vi "motor run execution.vi"(8 "error in":errorcluster, 10 "data":T3, 11 "Refnum Cluster Motor":T1) -> (0 "error out":errorcluster, 2 "Motor TextLog":string, 3 "Motor Log":string[][](array[string]))   [LabVIEW 2022 SP3]
uses:
  7f3f7f10-a4f1-45dc-94b5-7ca3060defcc.vi
  3e648d45-6e5c-4607-959b-4bd81591d8b7.vi
  3b4dbe33-a398-4ae1-98f2-0f6a12eff476.vi
  f93c375e-c4a4-4129-880d-4f6f32d70360.vi
  42315686-0e40-4c30-95d1-eb6a4dfe8554.vi
  62005152-647d-4142-ac27-8e0444444e4d.vi
  720007ab-8e7a-4def-9525-68d42a256be9.vi
  5550de12-40e6-485b-bfc0-db9a801049c2.vi
  3894978a-308b-403e-95e7-56de26c9271f.vi
  71392560-3ac6-4d43-9930-287395f3e7a2.vi
  pectus/control/Param Epics Cluster.ctl
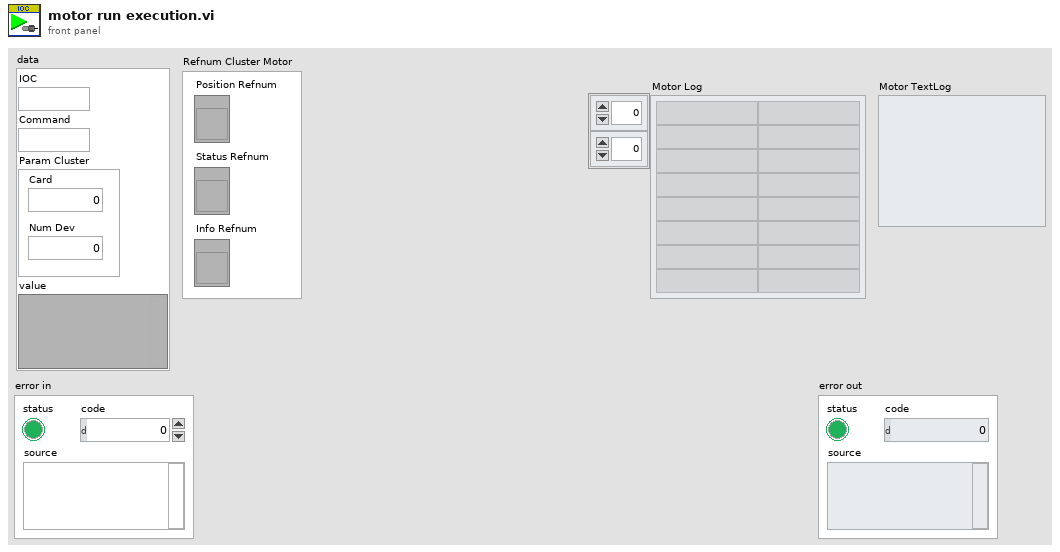
[diagram p1: front panel]
types:
  T1 = cluster{"Position Refnum":refnum<vi>, "Status Refnum":refnum<vi>, "Info Refnum":refnum<vi>}
  T2 = typedef "Param Epics Cluster.ctl" = cluster{"Card":u16, "Num Dev":u16}
  T3 = cluster{"IOC":string, "Command":string, "Param Cluster":T2, "value":variant}
  T4 = typedef "epics value.ctl" = cluster{"Record":string, "Value Out":variant}
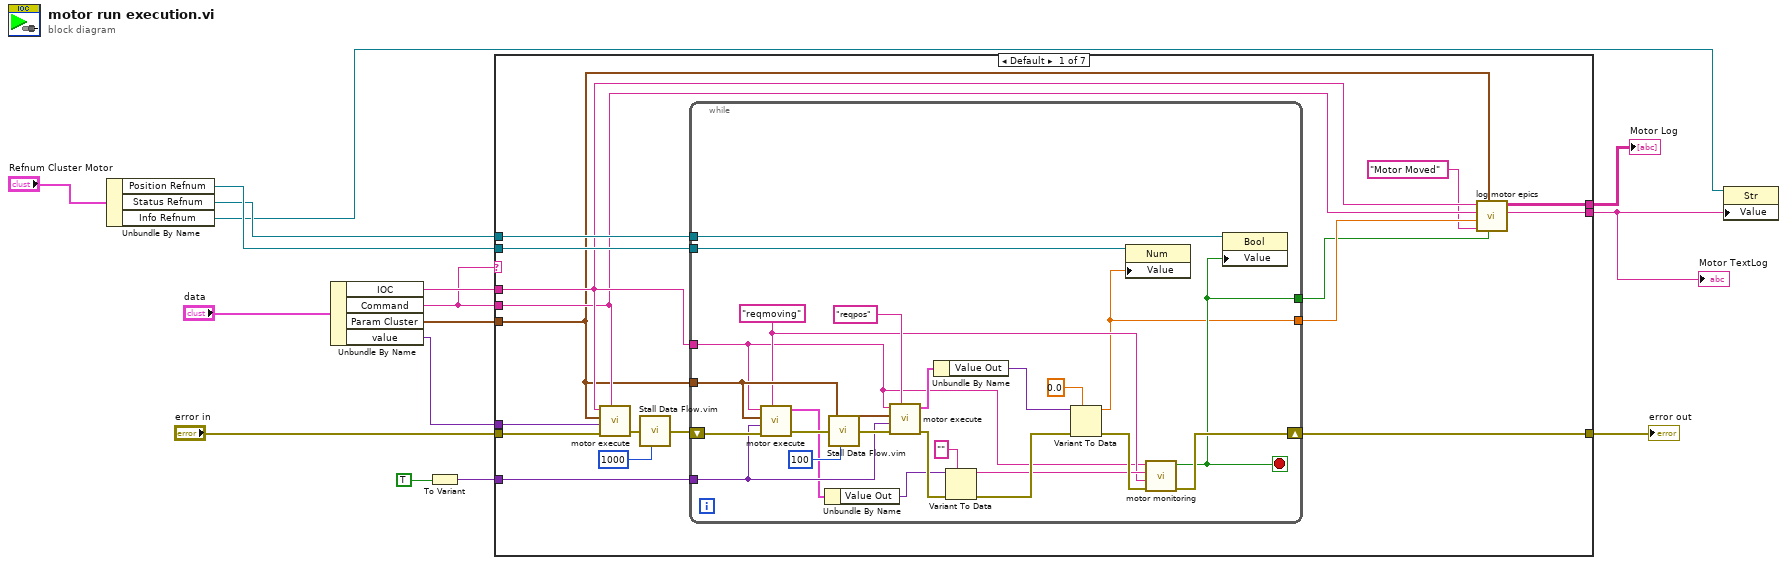
[diagram p0: block diagram]
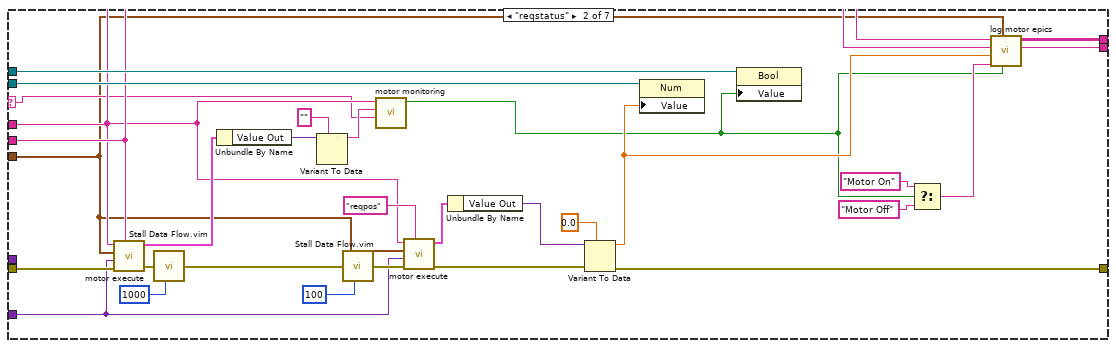
[diagram p2: hidden frame]
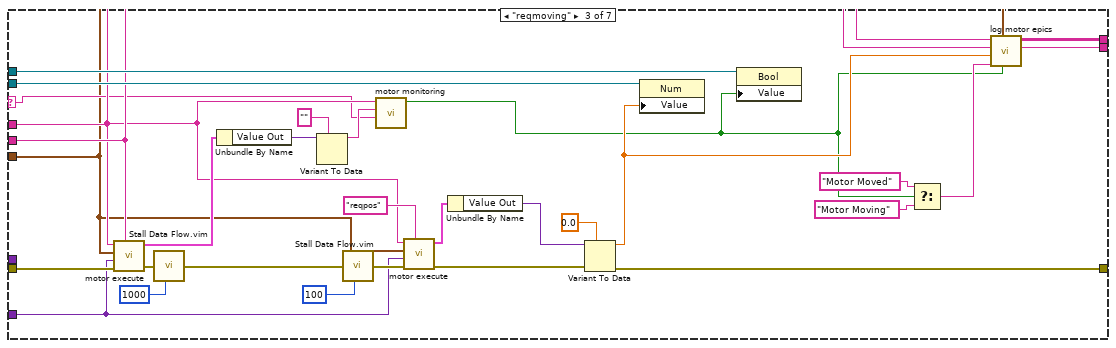
[diagram p3: hidden frame]
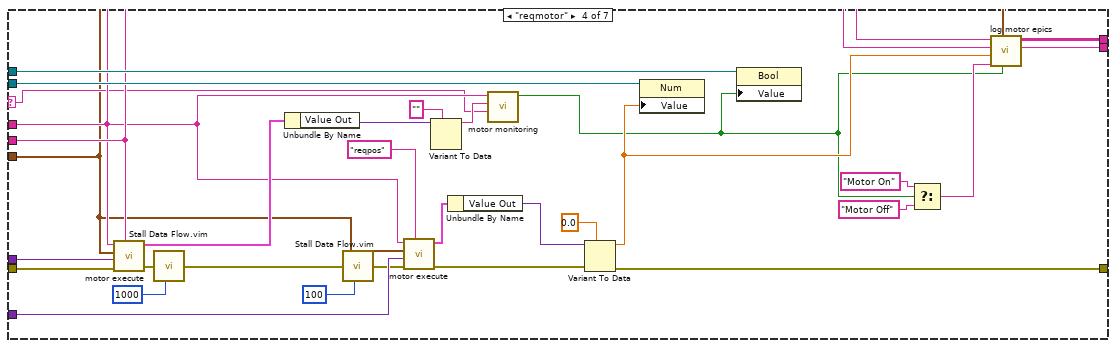
[diagram p4: hidden frame]
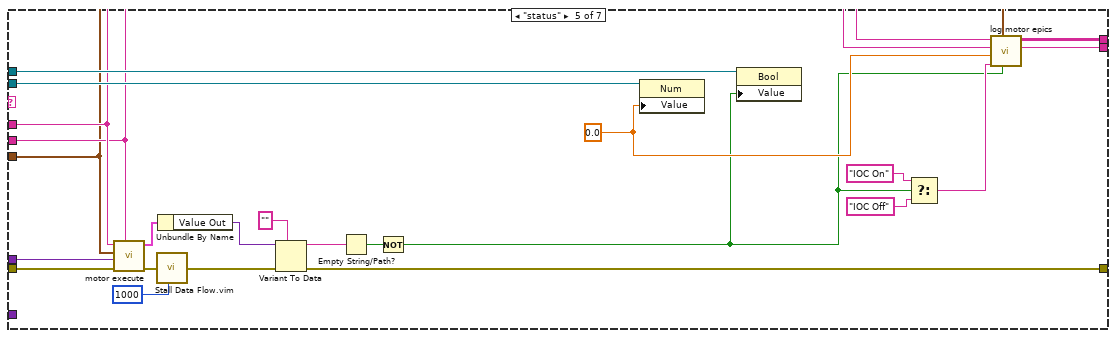
[diagram p5: hidden frame]
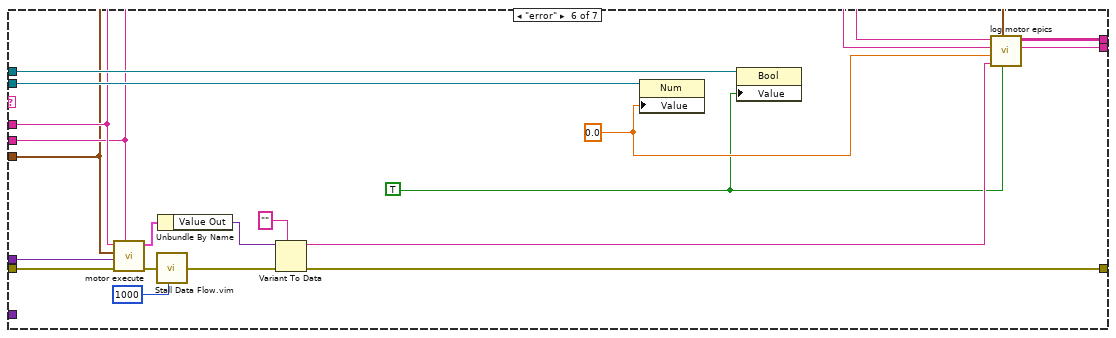
[diagram p6: hidden frame]
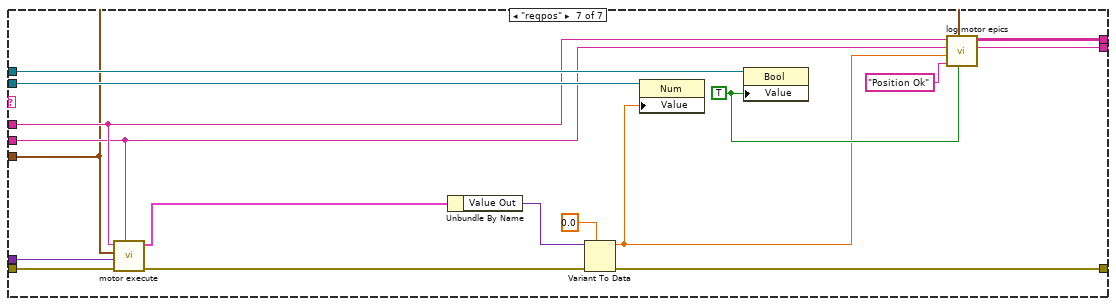
[diagram p7: hidden frame]
diagram:
  n1 = Unbundle By Name("Refnum Cluster Motor") -> ("Position Refnum"=w5:refnum<vi>, "Status Refnum"=w4:refnum<vi>, "Info Refnum"=w1:refnum<vi>)
  n2 = Unbundle By Name("data") -> ("IOC"=w13:string, "Command"=w7:string, "Param Cluster"=w14:T2, "value"=w11:variant)
  n3 = To Variant(anything=TRUE) -> (Variant=w15:variant)
  n4 = case shown="Default" w7 {
    selector: w7 -> [_ w59 w89 w118 _ _ _]
    tunnel: w15 -> [w29 w63 w93 w144 _ _ _]
    tunnel: w14 -> [w16 w57 w87 w117 w148 w171 w190]
    tunnel: w13 -> [w23 w62 w92 w120 w163 w182 w194]
    tunnel: w11 -> [w28 _ _ w143 w167 w186 w205]
    tunnel: w7 -> [w20 w78 w108 w137 w161 w180 w193]
    tunnel: "error in" -> [w27 w83 w113 w142 w166 w185 w204]
    tunnel: [w26 w82 w112 w141 w158 w177 w203] -> w8
    tunnel: w5 -> [w25 w81 w111 w140 w165 w184 w202]
    tunnel: w4 -> [w24 w80 w110 w139 w164 w183 w201]
    tunnel: [w19 w77 w107 w136 w160 w179 w197] -> w3
    tunnel: [w18 w76 w106 w135 w159 w178 w196] -> w2
    frame Default {
      n5 = call "motor execute.vi"("Command Motor"=w20, "error in"=w27, "Value"=w28, "Param Cluster"=w16, "IOC"=w23) -> ("error out"=w30:errorcluster)  [unwired: 3 in, 3 out]
      n6 = call "Stall Data Flow.vim"("value in"=w30, "milliseconds to wait"=u32 1000) -> ("value out"=w31:errorcluster)  [unwired: 1 out]
      n7 = while {
        shift-right: [w39] -> w26
        shift-left: w31 -> [w56]
        tunnel: w23 -> [w35]
        tunnel: w16 -> [w50]
        tunnel: w29 -> [w52]
        tunnel: w25 -> [w41]
        tunnel: w24 -> [w36]
        tunnel: [w34] -> w21
        tunnel: [w33] -> w22
        stop <- w34 stop-if-true
        w37 = "reqmoving"
        n8 = call "motor execute.vi"("Command Motor"=w37, "error in"=w56, "Value"=w52, "Param Cluster"=w50, "IOC"=w35) -> ("error out"=w55:errorcluster, "Data Value Out"=w43:T4)  [unwired: 3 in, 2 out]
        n9 = Unbundle By Name(w43) -> ("Value Out"=w42:variant)
        n10 = call "Stall Data Flow.vim"("value in"=w55, "milliseconds to wait"=u32 100) -> ("value out"=w53:errorcluster)  [unwired: 1 out]
        n11 = call "motor execute.vi"("Command Motor"="reqpos", "error in"=w53, "Value"=w52, "Param Cluster"=w50, "IOC"=w35) -> ("error out"=w46:errorcluster, "Data Value Out"=w47:T4)  [unwired: 3 in, 2 out]
        n12 = Unbundle By Name(w47) -> ("Value Out"=w49:variant)
        n13 = Variant To Data(error in=w46, type="", Variant=w42) -> (data=w38:string, error out=w45:errorcluster)
        n14 = Variant To Data(error in=w45, type=0.0, Variant=w49) -> (data=w33:dbl, error out=w40:errorcluster)
        n15 = property on="Property Node" class="Num"(reference=w41, "Value"=w33) -> ()  [unwired: 1 in, 2 out]
        n16 = call "motor monitoring.vi"("error in"=w40, "record"=w37, "Value"=w38, "IOC"=w35) -> ("error out"=w39:errorcluster, "Moved"=w34:bool)  [unwired: 6 in]
        n17 = property on="Property Node" class="Bool"(reference=w36, "Value"=w34) -> ()  [unwired: 1 in, 2 out]
      }
      n18 = call "log motor epics.vi"("status"=w21, "Param Cluster"=w16, "Info"="Motor Moved", "Position"=w22, "Command"=w20, "IOC"=w23) -> ("Motor TextLog"=w18:string, "Motor Log"=w19:string[][])  [unwired: 4 in]
    }
    frame "reqstatus" {
      n19 = call "motor execute.vi"("Command Motor"=w78, "error in"=w83, "Value"=w63, "Param Cluster"=w57, "IOC"=w62) -> ("error out"=w84:errorcluster, "Data Value Out"=w64:T4)  [unwired: 3 in, 2 out]
      n20 = call "Stall Data Flow.vim"("value in"=w84, "milliseconds to wait"=u32 1000) -> ("value out"=w85:errorcluster)  [unwired: 1 out]
      n21 = Unbundle By Name(w64) -> ("Value Out"=w65:variant)
      n22 = Variant To Data(type="", Variant=w65) -> (data=w60:string)  [unwired: 1 in, 1 out]
      n23 = call "Stall Data Flow.vim"("value in"=w85, "milliseconds to wait"=u32 100) -> ("value out"=w71:errorcluster)  [unwired: 1 out]
      n24 = call "motor monitoring.vi"("record"=w59, "Value"=w60, "IOC"=w62) -> ("Moved"=w58:bool)  [unwired: 7 in, 1 out]
      n25 = call "motor execute.vi"("Command Motor"="reqpos", "error in"=w71, "Value"=w63, "Param Cluster"=w57, "IOC"=w62) -> ("error out"=w66:errorcluster, "Data Value Out"=w67:T4)  [unwired: 3 in, 2 out]
      n26 = Unbundle By Name(w67) -> ("Value Out"=w69:variant)
      n27 = Variant To Data(error in=w66, type=0.0, Variant=w69) -> (data=w79:dbl, error out=w82:errorcluster)
      n28 = property on="Property Node" class="Num"(reference=w81, "Value"=w79) -> ()  [unwired: 1 in, 2 out]
      n29 = property on="Property Node" class="Bool"(reference=w80, "Value"=w58) -> ()  [unwired: 1 in, 2 out]
      n30 = Select(t="Motor On" ("Info"), s=w58, f="Motor Off" ("Info")) -> (s? t:f=w73:string)
      n31 = call "log motor epics.vi"("status"=w58, "Param Cluster"=w57, "Info"=w73, "Position"=w79, "Command"=w78, "IOC"=w62) -> ("Motor TextLog"=w76:string, "Motor Log"=w77:string[][])  [unwired: 4 in]
    }
    frame "reqmoving" {
      n32 = call "motor execute.vi"("Command Motor"=w108, "error in"=w113, "Value"=w93, "Param Cluster"=w87, "IOC"=w92) -> ("error out"=w114:errorcluster, "Data Value Out"=w94:T4)  [unwired: 3 in, 2 out]
      n33 = call "Stall Data Flow.vim"("value in"=w114, "milliseconds to wait"=u32 1000) -> ("value out"=w115:errorcluster)  [unwired: 1 out]
      n34 = Unbundle By Name(w94) -> ("Value Out"=w95:variant)
      n35 = Variant To Data(type="", Variant=w95) -> (data=w90:string)  [unwired: 1 in, 1 out]
      n36 = call "Stall Data Flow.vim"("value in"=w115, "milliseconds to wait"=u32 100) -> ("value out"=w101:errorcluster)  [unwired: 1 out]
      n37 = call "motor monitoring.vi"("record"=w89, "Value"=w90, "IOC"=w92) -> ("Moved"=w88:bool)  [unwired: 7 in, 1 out]
      n38 = call "motor execute.vi"("Command Motor"="reqpos", "error in"=w101, "Value"=w93, "Param Cluster"=w87, "IOC"=w92) -> ("error out"=w96:errorcluster, "Data Value Out"=w97:T4)  [unwired: 3 in, 2 out]
      n39 = Unbundle By Name(w97) -> ("Value Out"=w99:variant)
      n40 = Variant To Data(error in=w96, type=0.0, Variant=w99) -> (data=w109:dbl, error out=w112:errorcluster)
      n41 = property on="Property Node" class="Num"(reference=w111, "Value"=w109) -> ()  [unwired: 1 in, 2 out]
      n42 = property on="Property Node" class="Bool"(reference=w110, "Value"=w88) -> ()  [unwired: 1 in, 2 out]
      n43 = Select(t="Motor Moved" ("Info"), s=w88, f="Motor Moving" ("Info")) -> (s? t:f=w103:string)
      n44 = call "log motor epics.vi"("status"=w88, "Param Cluster"=w87, "Info"=w103, "Position"=w109, "Command"=w108, "IOC"=w92) -> ("Motor TextLog"=w106:string, "Motor Log"=w107:string[][])  [unwired: 4 in]
    }
    frame "reqmotor" {
      n45 = call "motor execute.vi"("Command Motor"=w137, "error in"=w142, "Value"=w143, "Param Cluster"=w117, "IOC"=w120) -> ("error out"=w145:errorcluster, "Data Value Out"=w124:T4)  [unwired: 3 in, 2 out]
      n46 = call "Stall Data Flow.vim"("value in"=w145, "milliseconds to wait"=u32 1000) -> ("value out"=w146:errorcluster)  [unwired: 1 out]
      n47 = Unbundle By Name(w124) -> ("Value Out"=w121:variant)
      n48 = call "Stall Data Flow.vim"("value in"=w146, "milliseconds to wait"=u32 100) -> ("value out"=w130:errorcluster)  [unwired: 1 out]
      n49 = call "motor execute.vi"("Command Motor"="reqpos", "error in"=w130, "Value"=w144, "Param Cluster"=w117, "IOC"=w120) -> ("error out"=w125:errorcluster, "Data Value Out"=w126:T4)  [unwired: 3 in, 2 out]
      n50 = Variant To Data(type="", Variant=w121) -> (data=w123:string)  [unwired: 1 in, 1 out]
      n51 = Unbundle By Name(w126) -> ("Value Out"=w128:variant)
      n52 = call "motor monitoring.vi"("record"=w118, "Value"=w123, "IOC"=w120) -> ("Moved"=w119:bool)  [unwired: 7 in, 1 out]
      n53 = Variant To Data(error in=w125, type=0.0, Variant=w128) -> (data=w138:dbl, error out=w141:errorcluster)
      n54 = property on="Property Node" class="Num"(reference=w140, "Value"=w138) -> ()  [unwired: 1 in, 2 out]
      n55 = property on="Property Node" class="Bool"(reference=w139, "Value"=w119) -> ()  [unwired: 1 in, 2 out]
      n56 = Select(t="Motor On" ("Info"), s=w119, f="Motor Off" ("Info")) -> (s? t:f=w132:string)
      n57 = call "log motor epics.vi"("status"=w119, "Param Cluster"=w117, "Info"=w132, "Position"=w138, "Command"=w137, "IOC"=w120) -> ("Motor TextLog"=w135:string, "Motor Log"=w136:string[][])  [unwired: 4 in]
    }
    frame "status" {
      w162 = 0.0
      n58 = call "motor execute.vi"("Command Motor"=w161, "error in"=w166, "Value"=w167, "Param Cluster"=w148, "IOC"=w163) -> ("error out"=w168:errorcluster, "Data Value Out"=w157:T4)  [unwired: 3 in, 2 out]
      n59 = call "Stall Data Flow.vim"("value in"=w168, "milliseconds to wait"=u32 1000) -> ("value out"=w169:errorcluster)  [unwired: 1 out]
      n60 = Unbundle By Name(w157) -> ("Value Out"=w156:variant)
      n61 = Variant To Data(error in=w169, type="", Variant=w156) -> (data=w154:string, error out=w158:errorcluster)
      n62 = Empty String/Path?(string/path=w154) -> (empty?=w153:bool)
      n63 = Not(x=w153) -> (.not. x?=w149:bool)
      n64 = property on="Property Node" class="Num"(reference=w165, "Value"=w162) -> ()  [unwired: 1 in, 2 out]
      n65 = property on="Property Node" class="Bool"(reference=w164, "Value"=w149) -> ()  [unwired: 1 in, 2 out]
      n66 = Select(t="IOC On" ("Info"), s=w149, f="IOC Off" ("Info")) -> (s? t:f=w150:string)
      n67 = call "log motor epics.vi"("status"=w149, "Param Cluster"=w148, "Info"=w150, "Position"=w162, "Command"=w161, "IOC"=w163) -> ("Motor TextLog"=w159:string, "Motor Log"=w160:string[][])  [unwired: 4 in]
    }
    frame "error" {
      w172 = TRUE
      w181 = 0.0
      n68 = call "motor execute.vi"("Command Motor"=w180, "error in"=w185, "Value"=w186, "Param Cluster"=w171, "IOC"=w182) -> ("error out"=w187:errorcluster, "Data Value Out"=w176:T4)  [unwired: 3 in, 2 out]
      n69 = call "Stall Data Flow.vim"("value in"=w187, "milliseconds to wait"=u32 1000) -> ("value out"=w188:errorcluster)  [unwired: 1 out]
      n70 = Unbundle By Name(w176) -> ("Value Out"=w175:variant)
      n71 = Variant To Data(error in=w188, type="", Variant=w175) -> (data=w173:string, error out=w177:errorcluster)
      n72 = property on="Property Node" class="Num"(reference=w184, "Value"=w181) -> ()  [unwired: 1 in, 2 out]
      n73 = property on="Property Node" class="Bool"(reference=w183, "Value"=w172) -> ()  [unwired: 1 in, 2 out]
      n74 = call "log motor epics.vi"("status"=w172, "Param Cluster"=w171, "Info"=w173, "Position"=w181, "Command"=w180, "IOC"=w182) -> ("Motor TextLog"=w178:string, "Motor Log"=w179:string[][])  [unwired: 4 in]
    }
    frame "reqpos" {
      w195 = TRUE ("Moved")
      n75 = call "motor execute.vi"("Command Motor"=w193, "error in"=w204, "Value"=w205, "Param Cluster"=w190, "IOC"=w194) -> ("error out"=w206:errorcluster, "Data Value Out"=w200:T4)  [unwired: 3 in, 2 out]
      n76 = Unbundle By Name(w200) -> ("Value Out"=w199:variant)
      n77 = Variant To Data(error in=w206, type=0.0, Variant=w199) -> (data=w192:dbl, error out=w203:errorcluster)
      n78 = property on="Property Node" class="Num"(reference=w202, "Value"=w192) -> ()  [unwired: 1 in, 2 out]
      n79 = property on="Property Node" class="Bool"(reference=w201, "Value"=w195) -> ()  [unwired: 1 in, 2 out]
      n80 = call "log motor epics.vi"("status"=w195, "Param Cluster"=w190, "Info"="Position Ok", "Position"=w192, "Command"=w193, "IOC"=w194) -> ("Motor TextLog"=w196:string, "Motor Log"=w197:string[][])  [unwired: 4 in]
    }
  }
  "error out" <- w8
  "Motor Log" <- w3
  "Motor TextLog" <- w2
  n81 = property on="Property Node" class="Str"(reference=w1, "Value"=w2) -> ()  [unwired: 1 in, 2 out]
